vi "Unpack Waveforms.vi"(11 "packed waveforms":dbl[][](array[numeric])) -> (3 "waveforms":waveform(dbl)[](array[waveform]))   [LabVIEW 2024, in "Dynamic Signal Acquisition (Interactive) UI.lvlib"]
uses:
  Dynamic Signal Acquisition (Interactive) UI.lvlib
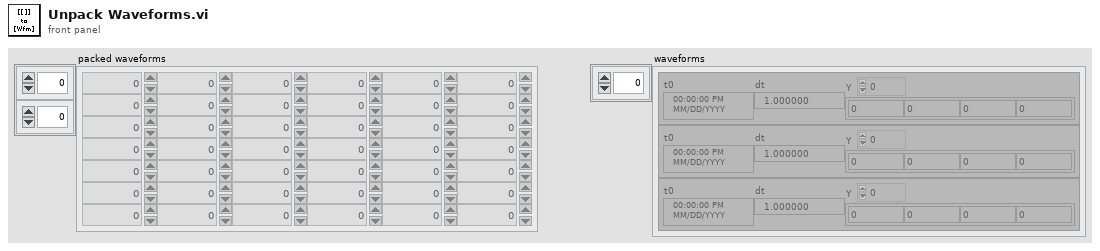
[diagram p1: front panel]
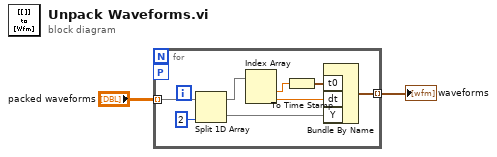
[diagram p0: block diagram]
diagram:
  n1 = for {
    workers-P: _ -> [_]
    tunnel: "packed waveforms" -> [w9] mode=indexing
    tunnel: [w3] -> w1 mode=indexing
    n2 = Split 1D Array(array=w9, index=2) -> (first subarray=w8:dbl[], second subarray=w7:dbl[])
    n3 = Index Array(array=w8) -> (element #1=w4:dbl, element #2=w6:dbl)  [unwired: 2 in]
    n4 = To Time Stamp(1:w4) -> (0:w5:timestamp)
    n5 = Bundle By Name("t0"=w5, "dt"=w6, "Y"=w7) -> (w3:waveform(dbl))  [unwired: 1 in]
  }
  "waveforms" <- w1
